vi "List Feeds and Packages in the SystemLink Repository.vi"() -> ()   [LabVIEW 2017]
doc: "This example shows how to open a connection to the SystemLink server and get a list of the feeds and packages in the SystemLink server's repository."
uses:
  SystemLink_Repo_API.lvlib
panel:
  in  "password":string
  in  "username":string
  in  "SystemLink server base URL":string="https://"
  out "List of all Packages in the SystemLink Repository":string[][](table)
  out "List of Feeds in the SystemLink Repository":string[](array[string])
  # "SystemLink Server"
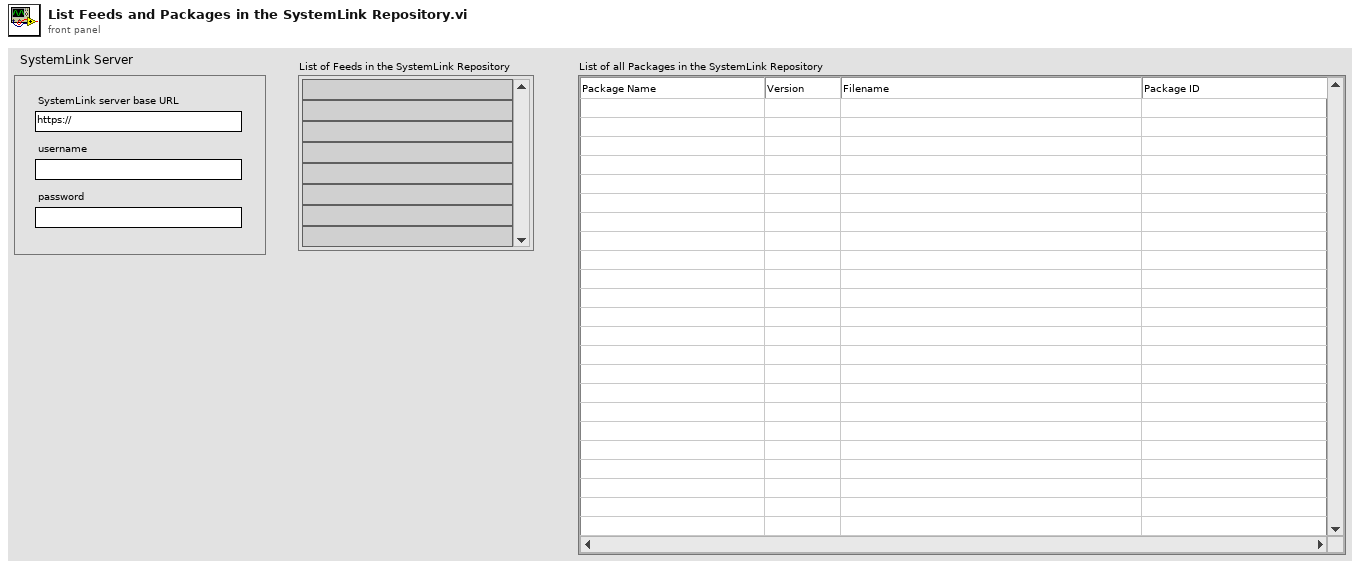
[diagram p1: front panel]
types:
  T1 = typedef "SystemLink_Repo_API.lvlib/systemlink repo.ctl" = cluster{"client handle out":T2, "SystemLink server base URL":string}
  T2 = typedef "LabVIEWHTTPClient.lvlib/ClientHandle.ctl" = refnum<k1>
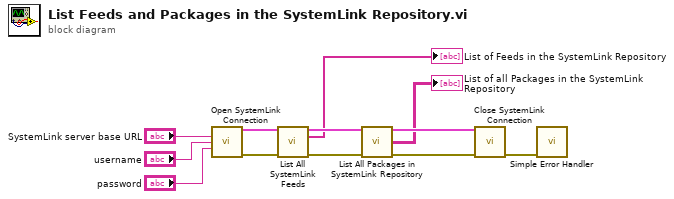
[diagram p0: block diagram]
diagram:
  n1 = call "Open SystemLink Connection.vi"("SystemLink server base URL"="SystemLink server base URL", "username"="username", "password"="password") -> ("SystemLink repo out"=w12:T1, "error out"=w11:errorcluster)  [unwired: 11 in]
  n2 = call "List All SystemLink Feeds.vi"("SystemLink repo in"=w12, "error in (no error)"=w11) -> ("SystemLink repo out"=w10:T1, "SystemLink Feed Names"=→"List of Feeds in the SystemLink Repository":string[], "error out"=w8:errorcluster)  [unwired: 10 in, 1 out]
  n3 = call "List All Packages in SystemLink Repository.vi"("SystemLink repo in"=w10, "error in (no error)"=w8) -> ("SystemLink repo out"=w9:T1, "packages"=→"List of all Packages in the SystemLink Repository":string[][], "error out"=w7:errorcluster)  [unwired: 11 in]
  n4 = call "Close SystemLink Connection.vi"("SystemLink repo in"=w9, "error in (no error)"=w7) -> ("error out"=w1:errorcluster)  [unwired: 13 in]
  n5 = call <vilib>:"Simple Error Handler.vi"("error in (no error)"=w1) -> ()  [unwired: 4 in, 5 out]
